vi "checkLaserStatus.vi"(8 "error in (no error)":errorcluster, 11 "Laser LED voltage":dbl[](array[numeric])) -> (0 "error out":errorcluster, 1 "Interlock open?":bool, 2 "Laser on?":bool, 3 "Mean voltage":dbl)   [LabVIEW 2024]
uses:
  <vilib>/Analysis/baseanly.llb/Mean (DBL).vi
  <vilib>/Analysis/NI_AALBase.lvlib
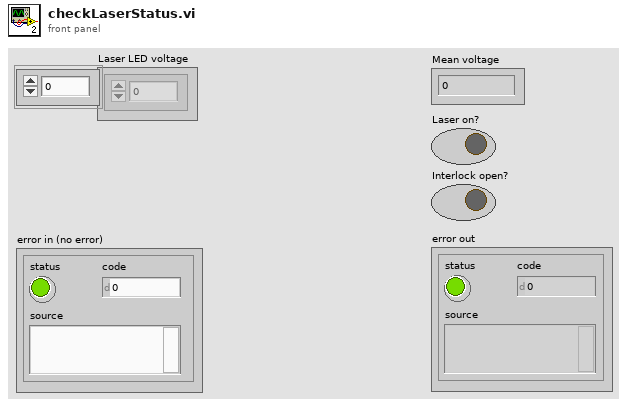
[diagram p1: front panel]
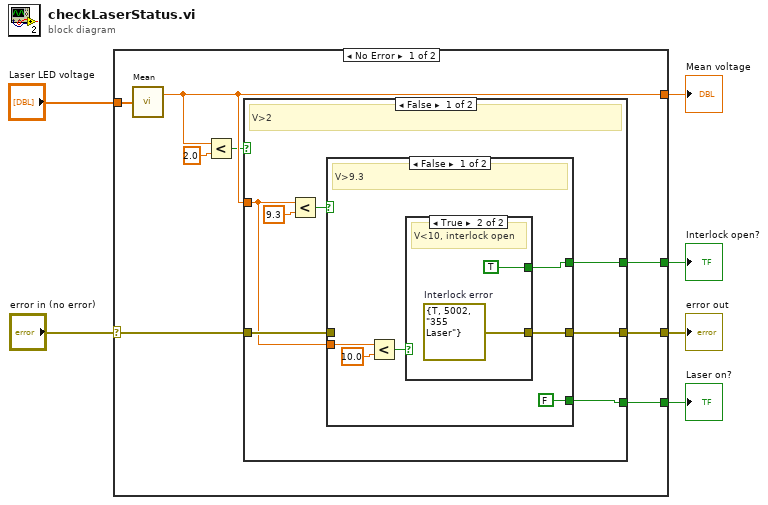
[diagram p0: block diagram]
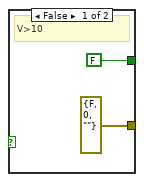
[diagram p2: hidden frame]
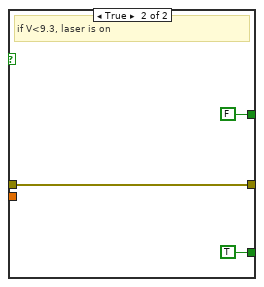
[diagram p3: hidden frame]
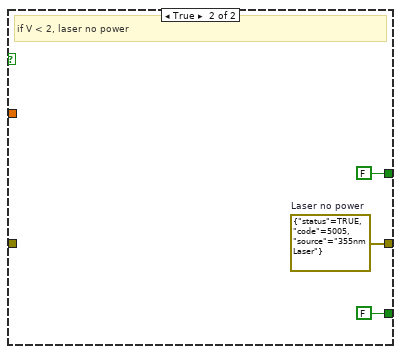
[diagram p4: hidden frame]
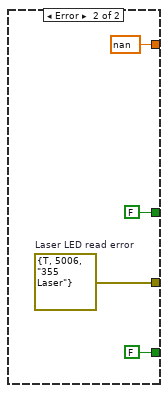
[diagram p5: hidden frame]
diagram:
  n1 = case shown="No Error" "error in (no error)" {
    selector: "error in (no error)" -> [w12 _]
    tunnel: [w14 FALSE] -> w2
    tunnel: [w13 w39] -> w3
    tunnel: [w10 nan] -> w5
    tunnel: "Laser LED voltage" -> [w11 _]
    tunnel: [w7 FALSE ("Blinking")] -> w1
    frame No Error {
      n2 = call-poly <vilib>:"Mean.vi"("X"=w11) -> ("mean"=w10:dbl)  [unwired: 1 out]
      n3 = Less?(x=w10, y=2.0) -> (x < y?=w8:bool)
      n4 = case shown="False" w8 {
        tunnel: [w19 FALSE] -> w14
        tunnel: w10 -> [w16 _]
        tunnel: w12 -> [w18 _]
        tunnel: [w17 w36] -> w13
        tunnel: [w15 FALSE ("Blinking")] -> w7
        frame False {
          # "V>2"
          n5 = Less?(x=w16, y=9.3) -> (x < y?=w20:bool)
          n6 = case shown="False" w20 {
            tunnel: [FALSE TRUE] -> w19
            tunnel: w18 -> [_ w33]
            tunnel: [w23 w33] -> w17
            tunnel: w16 -> [w26 _]
            tunnel: [w22 FALSE ("Blinking")] -> w15
            frame False {
              # "V>9.3"
              n7 = Less?(x=w26, y=10.0) -> (x < y?=w24:bool)
              n8 = case shown="True" w24 {
                tunnel: [errorcluster {"status"=FALSE, "code"=0, "source"=""} ("error out") w31] -> w23
                tunnel: [FALSE ("Blinking") TRUE ("Blinking")] -> w22
                frame False {
                  # "V>10"
                }
                frame True {
                  w31 = errorcluster {"status"=TRUE, "code"=5002, "source"="355 Laser"}  # Interlock error
                  # "V<10, interlock open"
                }
              }
            }
            frame True {
              # "if V<9.3, laser is on"
            }
          }
        }
        frame True {
          w36 = errorcluster {"status"=TRUE, "code"=5005, "source"="355nm Laser"}  # Laser no power
          # "if V < 2, laser no power"
        }
      }
    }
    frame Error {
      w39 = errorcluster {"status"=TRUE, "code"=5006, "source"="355 Laser"}  # Laser LED read error
    }
  }
  "Mean voltage" <- w5
  "error out" <- w3
  "Laser on?" <- w2
  "Interlock open?" <- w1
